vi "Display Array.vi"(0 "Timeout (5 seconds)":dbl=5.0, 1 "stop":bool, 2 "Array":dbl[](graph), 3 "Plot.Line Style":u8, 4 "Plot.Plot Interpolation":u8, 5 "Plot.Bar Plot Style":u8) -> ()   [LabVIEW 2012]
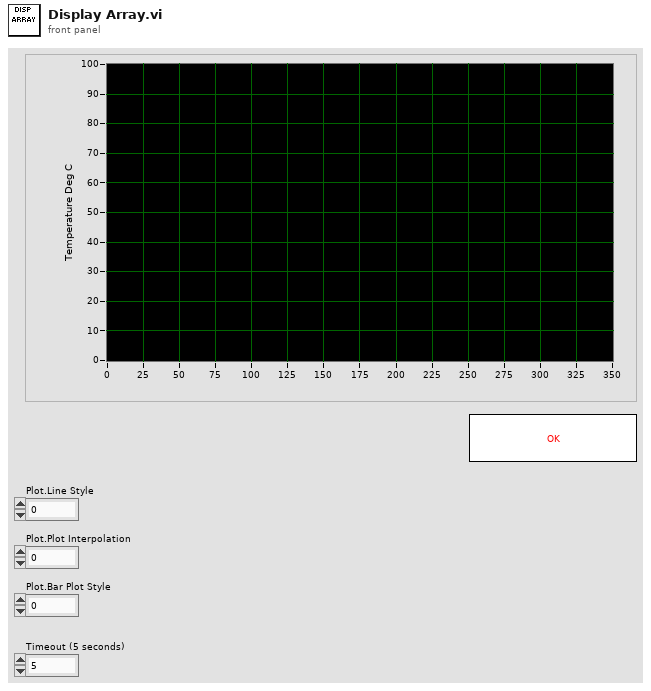
[diagram p1: front panel]
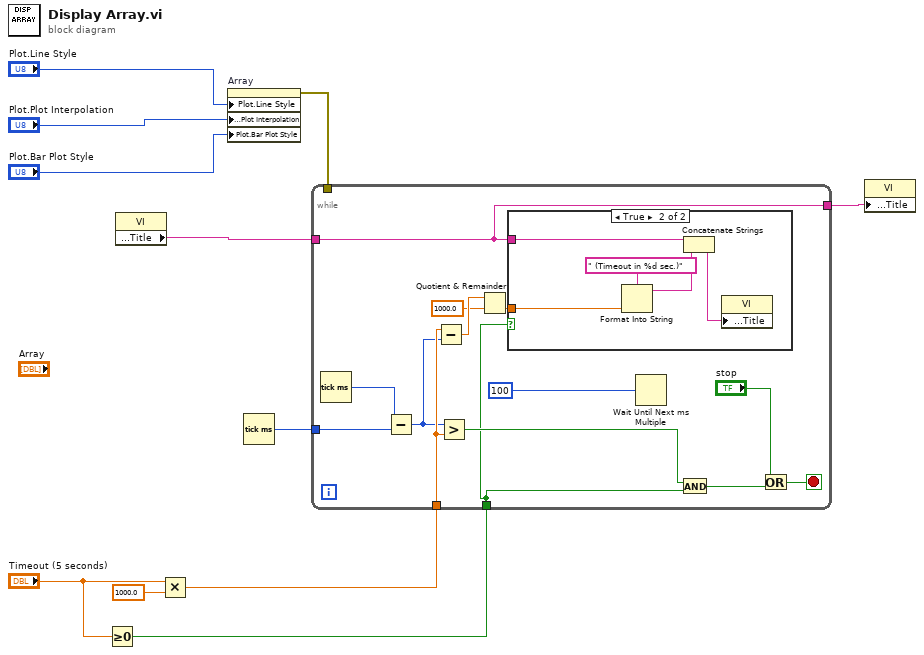
[diagram p0: block diagram]
diagram:
  n1 = Greater Or Equal To 0?(x="Timeout (5 seconds)") -> (x >= 0?=w4:bool)
  n2 = property class="VI"() -> ("Front Panel Window:Title"=w2:string)  [unwired: 2 in, 2 out]
  n3 = Multiply(x="Timeout (5 seconds)", y=1000.0) -> (x*y=w3:dbl)
  n4 = property on="Array" class="WFGraph (strict)"("Plot.Line Style"="Plot.Line Style", "Plot.Plot Interpolation"="Plot.Plot Interpolation", "Plot.Bar Plot Style"="Plot.Bar Plot Style") -> (error out=w8:errorcluster)  [unwired: 2 in, 1 out]
  n5 = Tick Count (ms)() -> (millisecond timer value=w7:u32)
  n6 = while {
    tunnel: w8 -> [_]
    tunnel: w7 -> [w23]
    tunnel: w4 -> [w18]
    tunnel: w3 -> [w17]
    tunnel: w2 -> [w12]
    tunnel: [w12] -> w1
    stop <- w21 stop-if-true
    n7 = Tick Count (ms)() -> (millisecond timer value=w24:u32)
    n8 = Subtract(x=w24, y=w23) -> (x-y=w16:u32)
    n9 = Subtract(x=w17, y=w16) -> (x-y=w15:dbl)
    n10 = Greater?(x=w16, y=w17) -> (0:w22:bool)
    n11 = Quotient & Remainder(x=w15, y=1000.0) -> (floor(x/y)=w13:dbl)  [unwired: 1 out]
    n12 = case shown="True" w18 {
      tunnel: w13 -> [_ w28]
      tunnel: w12 -> [_ w30]
      frame False {
        # "No Timeout don't need\nto update titlebar"
      }
      frame True {
        n13 = Format Into String(format string=" (Timeout in %d sec.)", w28) -> (resulting string=w26:string)  [unwired: 2 in, 1 out]
        n14 = Concatenate Strings(w30, w26) -> (w29:string)
        n15 = property class="VI"("Front Panel Window:Title"=w29) -> ()  [unwired: 2 in, 2 out]
      }
    }
    n16 = Wait Until Next ms Multiple(millisecond multiple=u32 100) -> ()  [unwired: 1 out]
    n17 = And(x=w22, y=w18) -> (x .and. y?=w20:bool)
    n18 = Or(x="stop", y=w20) -> (x .or. y?=w21:bool)
  }
  n19 = property class="VI"("Front Panel Window:Title"=w1) -> ()  [unwired: 2 in, 2 out]
